vi "cam_modpptest.vi"() -> ()   [LabVIEW 2013]
uses:
  <vilib>/userdefined/High Color/IMAQdx.ctl
  <vilib>/vision/Image Controls.llb/IMAQ Image.ctl
  <vilib>/vision/driver/NI_Vision_Acquisition_Software.lvlib
panel:
  out "Image":T1(plugin-control)
  out "error out":errorcluster
  out "Session Out":T2
  in  "error in":errorcluster
  out "Image reference":T1
  in  "Camera":T2="cam0"
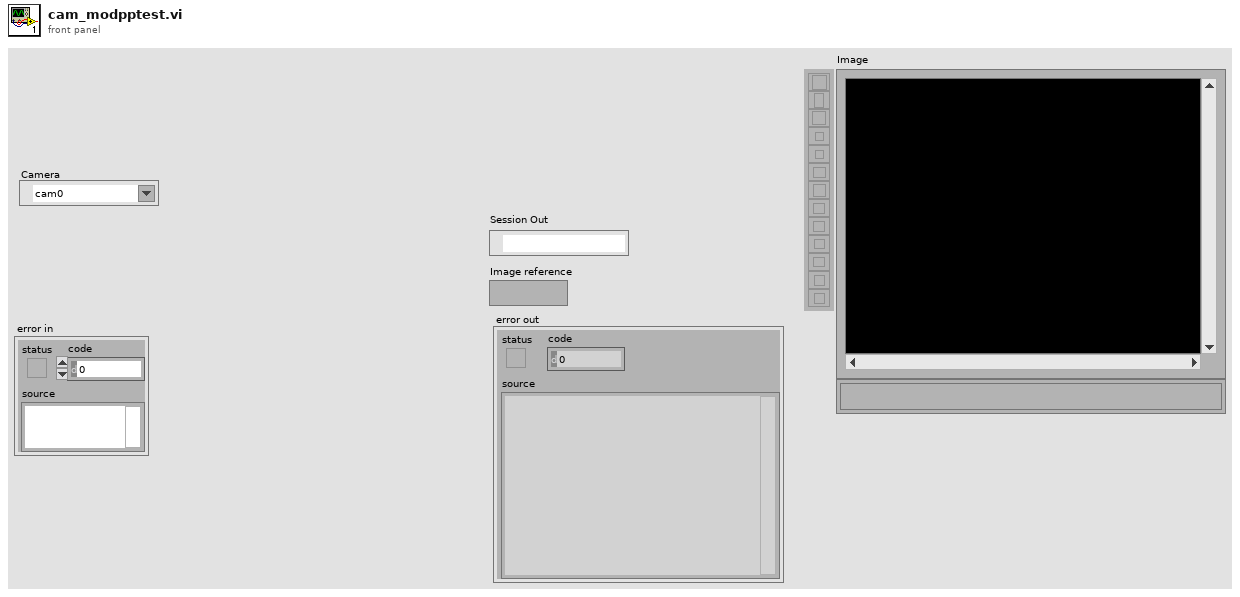
[diagram p1: front panel]
types:
  T1 = typedef "IMAQ Image.ctl" = refnum<image>
  T2 = typedef "IMAQdx.ctl" = refnum<k21>
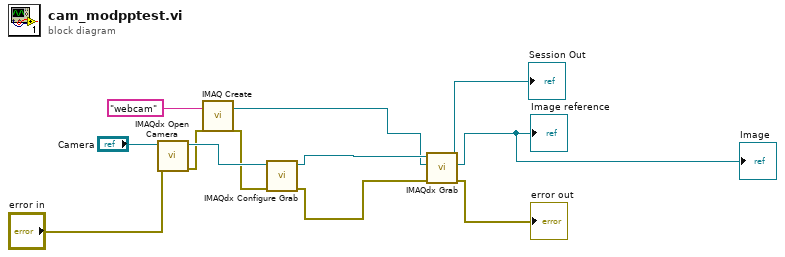
[diagram p0: block diagram]
diagram:
  n1 = call <vilib>:"IMAQdx Open Camera.vi"("error in"="error in", "Session In"="Camera") -> ("error out"=w9:errorcluster, "Session Out"=w12:T2)  [unwired: 8 in]
  n2 = call "IMAQ Create"("Image Name"="webcam", "error in (no error)"=w9) -> ("New Image"=w5:T1, "error out"=w8:errorcluster)  [unwired: 3 in]
  n3 = call <vilib>:"IMAQdx Configure Grab.vi"("error in"=w8, "Session In"=w12) -> ("error out"=w3:errorcluster, "Session Out"=w6:T2)  [unwired: 8 in]
  n4 = call <vilib>:"IMAQdx Grab.vi"("error in"=w3, "Image In"=w5, "Session In"=w6) -> ("error out"=→"error out":errorcluster, "Image Out"=→"Image reference" →"Image":T1, "Session Out"=→"Session Out":T2)  [unwired: 5 in, 1 out]
